vi "getCameraSubData.vi"(7 "Refnum in":T1, 8 "error in (no error)":errorcluster, 9 "VDim":i32, 10 "HDim":i32, 11 "arrayIn":u32[](array[numeric])) -> (0 "error out":errorcluster, 2 "arrayOut":u32[](array[numeric]), 5 "Refnum out":T1)   [LabVIEW 2016]
uses:
  <vilib>/vision/Image Controls.llb/IMAQ Image.ctl
  cameraLibrary/build-cameraLibrary/labview-import/cameraLibrary.lvlib
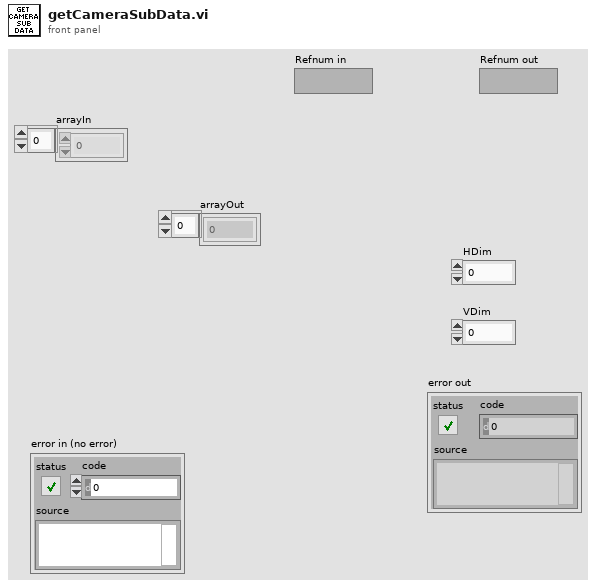
[diagram p1: front panel]
types:
  T1 = typedef "IMAQ Image.ctl" = refnum<image>
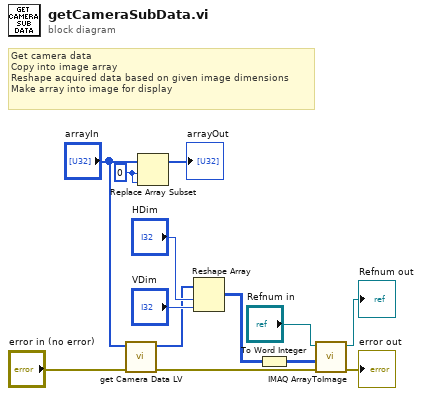
[diagram p0: block diagram]
diagram:
  w1 = u32 0 ("index")
  # "Get camera data\nCopy into image array\nReshape acquired data based on given image dimensions\nMake array into image for display"
  n1 = call "get Camera Data LV.vi"("error in (no error)"="error in (no error)", "dataIn"="arrayIn") -> ("error out"=w4:errorcluster, "dataOut"=w5:u32[])  [unwired: 8 in]
  n2 = Replace Array Subset(array="arrayIn", new element=w1, index=w1) -> (→"arrayOut":u32[])
  n3 = Reshape Array(w5, "HDim", "VDim") -> (w3:u32[][])
  n4 = To Word Integer(number=w3) -> (16bit integer=w2:i16[][])
  n5 = call "IMAQ ArrayToImage"("error in (no error)"=w4, "Image Pixels (I16)"=w2, "Image"="Refnum in") -> ("error out"=→"error out":errorcluster, "Image Out"=→"Refnum out":T1)  [unwired: 7 in]
